vi "VIPM Get Package_LabVIEW_Version.vi"(11 "XML File Path":path) -> (3 "Package_LabVIEW_Version":string)   [LabVIEW 2019, in "Build.lvlib"]
uses:
  Build.lvlib
  <vilib>/xml/Close Reference(Node).vi
  <resource>/objmgr/DOMUserDefRef.rc
  <vilib>/xml/NI_XML.lvlib
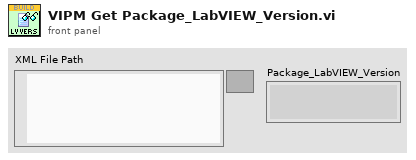
[diagram p1: front panel]
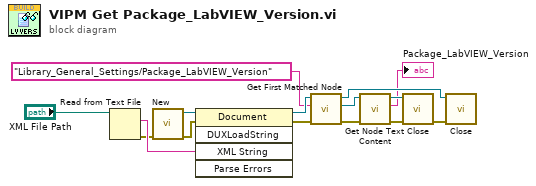
[diagram p0: block diagram]
diagram:
  n1 = Read from Text File(file (use dialog)="XML File Path") -> (text=w13:string, error out=w7:errorcluster)  [unwired: 3 in, 2 out]
  n2 = call <vilib>:"New.vi"("error in (no error)"=w7) -> ("error out"=w6:errorcluster, "DOM document out"=w14:refnum<k20>)  [unwired: 7 in]
  n3 = invoke class="Document" method="DUXLoadString"(reference=w14, error in=w6, "XML String"=w13) -> (reference out=w12:refnum<k20>, error out=w5:errorcluster)  [unwired: 2 in, 3 out]
  n4 = call <vilib>:"Get First Matched Node.vi"("error in (no error)"=w5, "XPath expression"="Library_General_Settings/Package_LabVIEW_Version", "node in"=w12) -> ("error out"=w4:errorcluster, "node result"=w10:refnum<k20>, "node out"=w11:refnum<k20>)  [unwired: 6 in]
  n5 = call <vilib>:"Get Node Text Content.vi"("error in (no error)"=w4, "node in"=w10) -> ("error out"=w3:errorcluster, "node text"=→"Package_LabVIEW_Version":string, "node out"=w9:refnum<k20>)  [unwired: 7 in]
  n6 = call-poly <vilib>:"Close.vi"("error in (no error)"=w3, "node"=w9) -> ("error out"=w2:errorcluster)  [unwired: 7 in]
  n7 = call-poly <vilib>:"Close.vi"("error in (no error)"=w2, "node"=w11) -> ()  [unwired: 7 in, 1 out]
